vi "Reset Table.vi"(8 "error in (no error)":errorcluster, 11 "Result Table.lvclass":refnum<class "Result Table.lvclass">) -> (0 "error out":errorcluster, 3 "Result Table":refnum<class "Result Table.lvclass">)   [LabVIEW 2020, in "Result Table.lvclass"]
uses:
  Result Table.lvclass
  Private/TypeDefs/Table Columns.ctl
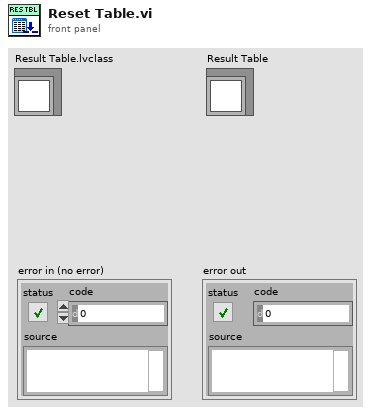
[diagram p1: front panel]
types:
  T1 = typedef "Result Table.lvclass/Table Columns.ctl" = u16
  T2 = typedef "Result Table.lvclass/Results.ctl" = cluster{"Method Count":u32, "Executed Methods":u32, "Passed Methods":u32, "Failed Methods":u32, "Method Errors":u32, "Skipped Method":u32}
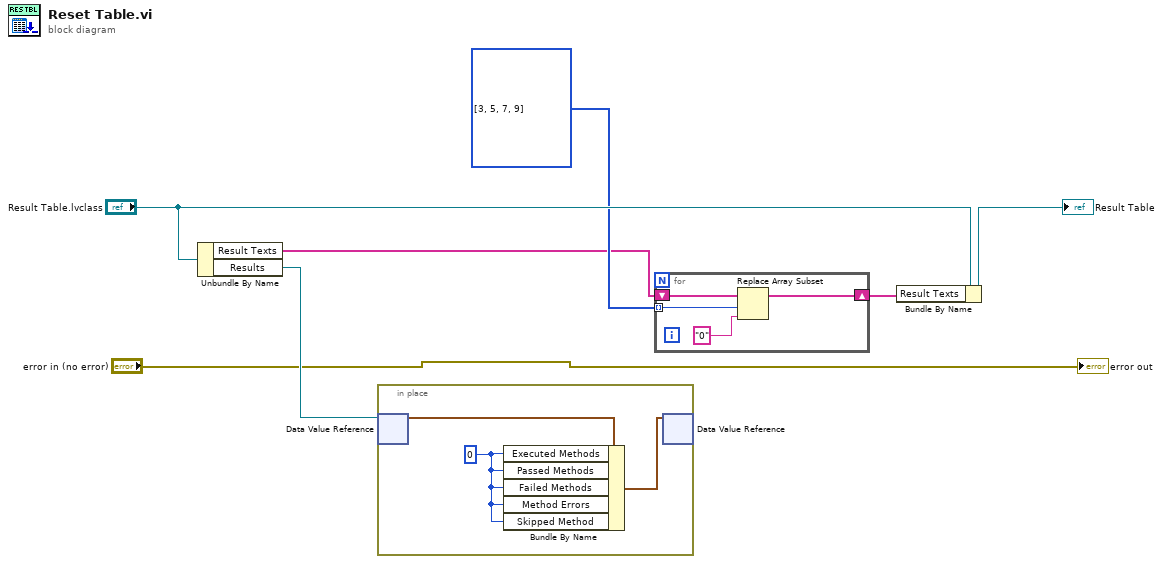
[diagram p0: block diagram]
diagram:
  w5 = T1[] [3, 5, 7, 9] items=["Last run:"=1, "Passed:"=3, "Failed:"=5, "Errors:"=7, "Skipped"=9]
  n1 = Unbundle By Name("Result Table.lvclass") -> ("Result Texts"=w4:string[], "Results"=w6:refnum<data-value>)
  n2 = in-place {
    w9 = u32 0 ("Method Count")
    n3 = in-place-dvr #1(w6) -> (w10:T2)  [unwired: 1 out]
    n4 = Bundle By Name(cluster=w10, "Executed Methods"=w9, "Passed Methods"=w9, "Failed Methods"=w9, "Method Errors"=w9, "Skipped Method"=w9) -> (w8:T2)
    n5 = in-place-dvr #1(w8) -> ()  [unwired: 2 out]
  }
  n6 = for {
    shift-right: [w12] -> w1
    shift-left: w4 -> [w14]
    tunnel: w5 -> [w11] mode=indexing
    n7 = Replace Array Subset(array=w14, new element="0" ("new element/subarray"), index=w11) -> (w12:string[])
  }
  n8 = Bundle By Name(cluster="Result Table.lvclass", "Result Texts"=w1) -> (→"Result Table":refnum<class "Result Table.lvclass">)
  "error out" <- "error in (no error)"
